vi "Create String Content.vi"(4 "encoding (ASCII)":refnum<k24>, 5 "HttpContent_String in":refnum<class "HttpContent_String.lvclass">, 6 "ContentType (text/plain)":T1="text/plain", 8 "error in (no error)":errorcluster, 11 "Content":string) -> (0 "error out":errorcluster, 3 "HttpContent_String out":refnum<class "HttpContent_String.lvclass">)   [LabVIEW 2018, in "LabVIEWHTTPClient_NET.lvlib" / "HttpContent_String.lvclass"]
uses:
  HttpContent_String.lvclass
  C:/Viviota/Projects/R&D/LabVIEW_HTTP_REST_NET/HttpContent/HttpContent.lvclass
  Types/ContentType.ctl
  System.Net.Http
  HttpContent/HttpContent.lvclass
  LabVIEWHTTPClient_NET/LabVIEWHTTPClient_NET.lvlib
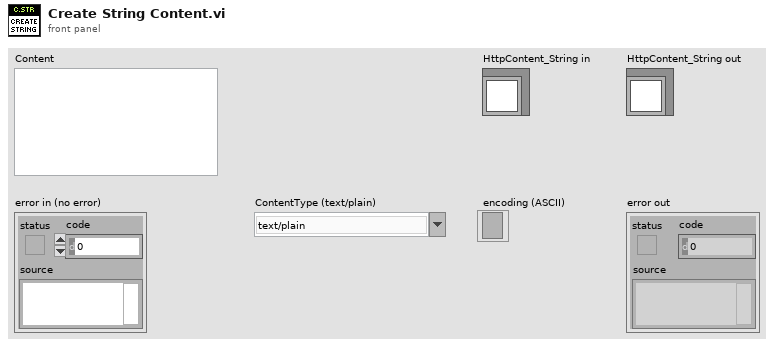
[diagram p1: front panel]
types:
  T1 = typedef "LabVIEWHTTPClient_NET.lvlib/ContentType.ctl" = string
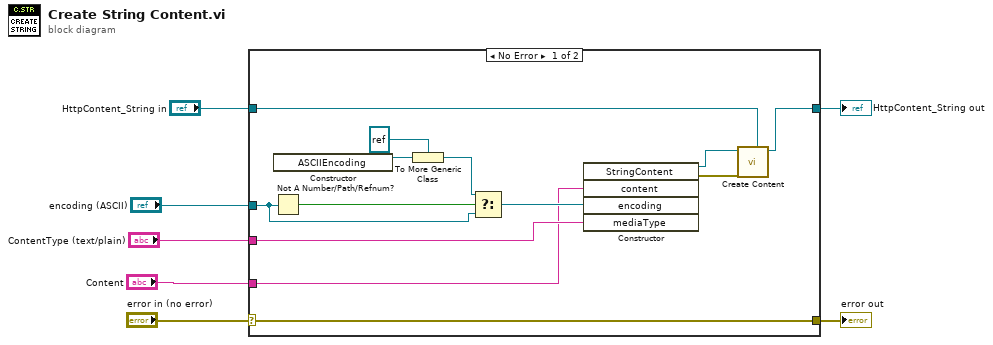
[diagram p0: block diagram]
diagram:
  n1 = case shown="No Error" "error in (no error)" {
    selector: "error in (no error)" -> [w20 w22]
    tunnel: [w20 w22] -> w6
    tunnel: [w18 w21] -> w4
    tunnel: "HttpContent_String in" -> [w19 w21]
    tunnel: "encoding (ASCII)" -> [w10 _]
    tunnel: "ContentType (text/plain)" -> [w15 _]
    tunnel: "Content" -> [w8 _]
    frame No Error {
      n2 = Not A Number/Path/Refnum?(number/path/refnum=w10) -> (NaN/Path/Refnum?=w14:bool)
      n3 = constructor class="ASCIIEncoding"() -> (reference out=w13:refnum<k24>)  [unwired: 3 in, 2 out]
      n4 = To More Generic Class(target class=refnum<k24> refnum ("encoding"), reference=w13) -> (generic class reference=w12:refnum<k24>)
      n5 = Select(t=w12, s=w14, f=w10) -> (s? t:f=w9:refnum<k24>)
      n6 = constructor class="StringContent"("content"=w8, "encoding"=w9, "mediaType"=w15) -> (reference out=w16:refnum<k24>, error out=w17:errorcluster)  [unwired: 3 in, 4 out]
      n7 = call "Create Content.vi"("HttpContent in"=w19, "error in (no error)"=w17, "NET_HttpContent"=w16) -> ("HttpContent out"=w18:refnum<class "HttpContent_String.lvclass">)  [unwired: 7 in, 1 out]
    }
    frame Error {
    }
  }
  "error out" <- w6
  "HttpContent_String out" <- w4
